vi "УУ.vi"(7 "Func":T1) -> (2 "Read":bool, 3 "Exec":bool, 4 "SelInp":bool, 6 "Wr":bool, 8 "SelOp":bool, 10 "ALU func":T1, 14 "Cread":bool, 15 "ClearAcc":bool)   [LabVIEW 2013]
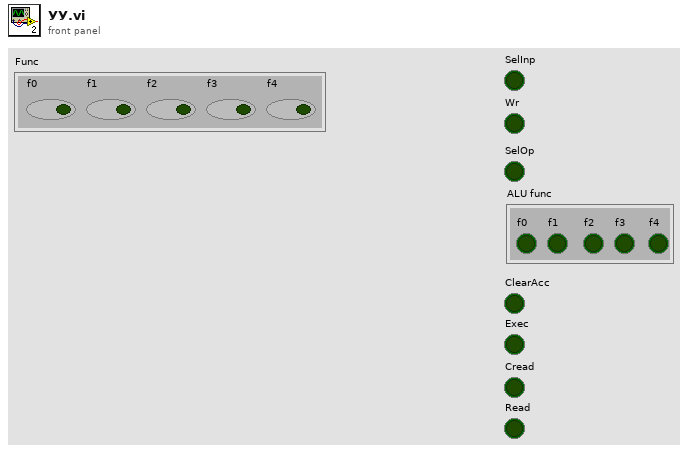
[diagram p1: front panel]
types:
  T1 = cluster{"f0":bool, "f1":bool, "f2":bool, "f3":bool, "f4":bool}
  T2 = cluster{bool, bool, bool, cluster{bool, bool, bool, bool, bool}, bool, bool, bool, bool}
  T3 = cluster{"SelInp":bool, "Wr":bool, "SelOp":bool, "ALU func":cluster{"f0":bool, "f1":bool, "f2":bool, "f3":bool, "f4":bool}, "ClearAcc":bool, "Exec":bool, "Cread":bool, "Read":bool}
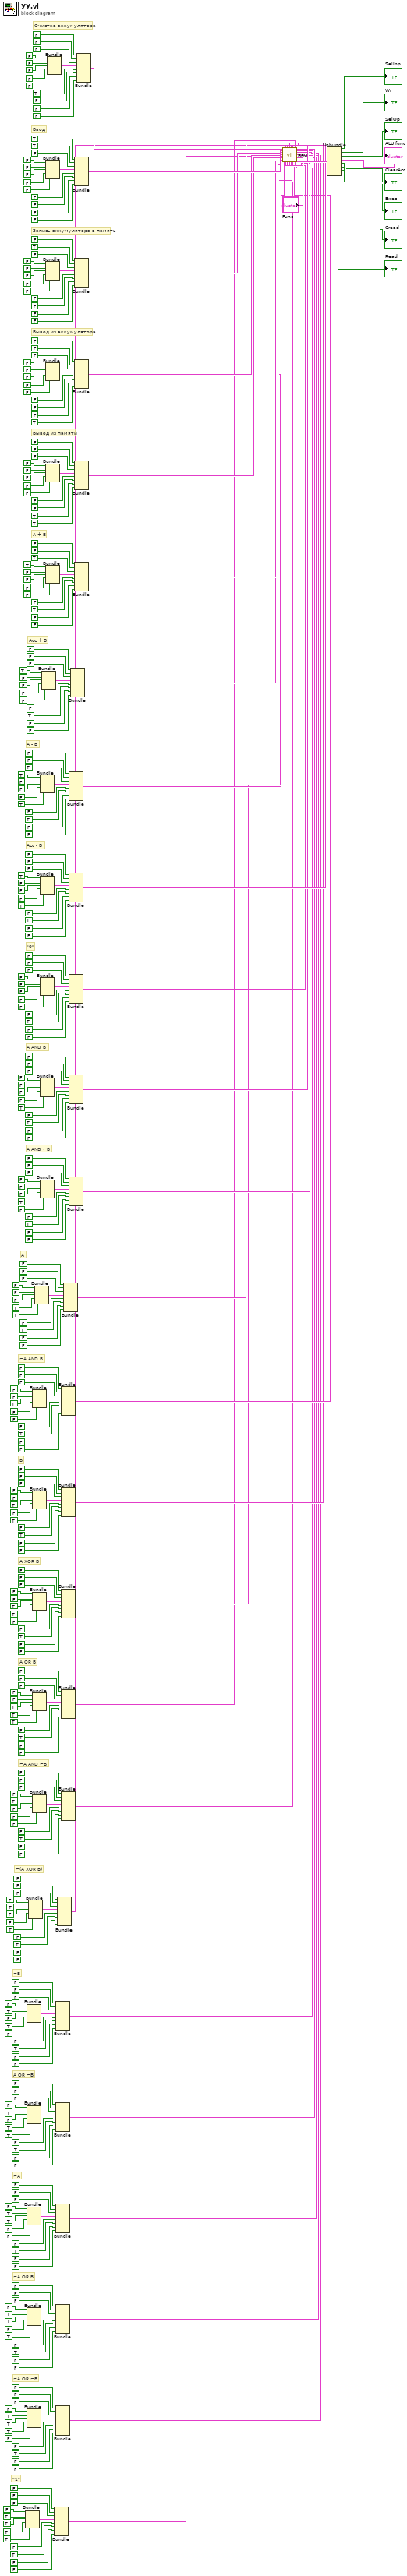
[diagram p0: block diagram]
diagram:
  # "\"1\""
  # "~A OR ~B"
  # "~A OR B"
  # "~A"
  # "A OR ~B"
  # "~B"
  # "~(A XOR B)"
  # "~A AND ~B"
  # "A OR B"
  # "A XOR B"
  # "B"
  # "~A AND B"
  # "A"
  # "A AND ~B"
  # "A AND B"
  # "\"0\""
  # "Acc - B"
  # "A - B"
  # "Acc + B"
  # "A + B"
  # "Вывод из памяти"
  # "Вывод из аккумулятора"
  # "Запись аккумулятора в память"
  # "Ввод"
  # "Очистка аккумулятора"
  n1 = Bundle(FALSE, TRUE, TRUE, TRUE, TRUE) -> (w30:cluster{bool, bool, bool, bool, bool})  [unwired: 1 in]
  n2 = Bundle(FALSE, TRUE, FALSE, TRUE, FALSE) -> (w95:cluster{bool, bool, bool, bool, bool})  [unwired: 1 in]
  n3 = Bundle(FALSE, TRUE, FALSE, TRUE, TRUE) -> (w82:cluster{bool, bool, bool, bool, bool})  [unwired: 1 in]
  n4 = Bundle(FALSE, TRUE, TRUE, FALSE, FALSE) -> (w69:cluster{bool, bool, bool, bool, bool})  [unwired: 1 in]
  n5 = Bundle(FALSE, TRUE, TRUE, FALSE, TRUE) -> (w56:cluster{bool, bool, bool, bool, bool})  [unwired: 1 in]
  n6 = Bundle(FALSE, TRUE, TRUE, TRUE, FALSE) -> (w43:cluster{bool, bool, bool, bool, bool})  [unwired: 1 in]
  n7 = Bundle(FALSE, TRUE, FALSE, FALSE, TRUE) -> (w108:cluster{bool, bool, bool, bool, bool})  [unwired: 1 in]
  n8 = Bundle(FALSE, FALSE, TRUE, FALSE, FALSE) -> (w173:cluster{bool, bool, bool, bool, bool})  [unwired: 1 in]
  n9 = Bundle(FALSE, FALSE, TRUE, FALSE, TRUE) -> (w160:cluster{bool, bool, bool, bool, bool})  [unwired: 1 in]
  n10 = Bundle(FALSE, FALSE, TRUE, TRUE, FALSE) -> (w147:cluster{bool, bool, bool, bool, bool})  [unwired: 1 in]
  n11 = Bundle(FALSE, FALSE, TRUE, TRUE, TRUE) -> (w134:cluster{bool, bool, bool, bool, bool})  [unwired: 1 in]
  n12 = Bundle(FALSE, TRUE, FALSE, FALSE, FALSE) -> (w121:cluster{bool, bool, bool, bool, bool})  [unwired: 1 in]
  n13 = Bundle(FALSE, FALSE, FALSE, TRUE, TRUE) -> (w186:cluster{bool, bool, bool, bool, bool})  [unwired: 1 in]
  n14 = Bundle(TRUE, FALSE, FALSE, FALSE, TRUE) -> (w251:cluster{bool, bool, bool, bool, bool})  [unwired: 1 in]
  n15 = Bundle(TRUE, FALSE, FALSE, FALSE, TRUE) -> (w238:cluster{bool, bool, bool, bool, bool})  [unwired: 1 in]
  n16 = Bundle(FALSE, FALSE, FALSE, FALSE, FALSE) -> (w225:cluster{bool, bool, bool, bool, bool})  [unwired: 1 in]
  n17 = Bundle(FALSE, FALSE, FALSE, FALSE, TRUE) -> (w212:cluster{bool, bool, bool, bool, bool})  [unwired: 1 in]
  n18 = Bundle(FALSE, FALSE, FALSE, TRUE, FALSE) -> (w199:cluster{bool, bool, bool, bool, bool})  [unwired: 1 in]
  n19 = Bundle(TRUE, FALSE, FALSE, FALSE, FALSE) -> (w264:cluster{bool, bool, bool, bool, bool})  [unwired: 1 in]
  n20 = Bundle(FALSE, FALSE, FALSE, FALSE, FALSE) -> (w329:cluster{bool, bool, bool, bool, bool})  [unwired: 1 in]
  n21 = Bundle(FALSE, FALSE, FALSE, FALSE, FALSE) -> (w316:cluster{bool, bool, bool, bool, bool})  [unwired: 1 in]
  n22 = Bundle(FALSE, FALSE, FALSE, FALSE, FALSE) -> (w303:cluster{bool, bool, bool, bool, bool})  [unwired: 1 in]
  n23 = Bundle(FALSE, FALSE, FALSE, FALSE, FALSE) -> (w290:cluster{bool, bool, bool, bool, bool})  [unwired: 1 in]
  n24 = Bundle(TRUE, FALSE, FALSE, FALSE, FALSE) -> (w277:cluster{bool, bool, bool, bool, bool})  [unwired: 1 in]
  n25 = Bundle(FALSE, FALSE, FALSE, FALSE, FALSE) -> (w342:cluster{bool, bool, bool, bool, bool})  [unwired: 1 in]
  n26 = Bundle(FALSE, FALSE, FALSE, w30, FALSE, TRUE, FALSE, FALSE) -> (w1:T2)  [unwired: 1 in]
  n27 = Bundle(FALSE, FALSE, FALSE, w95, FALSE, TRUE, FALSE, FALSE) -> (w6:T2)  [unwired: 1 in]
  n28 = Bundle(FALSE, FALSE, FALSE, w82, FALSE, TRUE, FALSE, FALSE) -> (w5:T2)  [unwired: 1 in]
  n29 = Bundle(FALSE, FALSE, FALSE, w69, FALSE, TRUE, FALSE, FALSE) -> (w4:T2)  [unwired: 1 in]
  n30 = Bundle(FALSE, FALSE, FALSE, w56, FALSE, TRUE, FALSE, FALSE) -> (w3:T2)  [unwired: 1 in]
  n31 = Bundle(FALSE, FALSE, FALSE, w43, FALSE, TRUE, FALSE, FALSE) -> (w2:T2)  [unwired: 1 in]
  n32 = Bundle(FALSE, FALSE, FALSE, w108, FALSE, TRUE, FALSE, FALSE) -> (w7:T2)  [unwired: 1 in]
  n33 = Bundle(FALSE, FALSE, FALSE, w173, FALSE, TRUE, FALSE, FALSE) -> (w12:T2)  [unwired: 1 in]
  n34 = Bundle(FALSE, FALSE, FALSE, w160, FALSE, TRUE, FALSE, FALSE) -> (w11:T2)  [unwired: 1 in]
  n35 = Bundle(FALSE, FALSE, FALSE, w147, FALSE, TRUE, FALSE, FALSE) -> (w10:T2)  [unwired: 1 in]
  n36 = Bundle(FALSE, FALSE, FALSE, w134, FALSE, TRUE, FALSE, FALSE) -> (w9:T2)  [unwired: 1 in]
  n37 = Bundle(FALSE, FALSE, FALSE, w121, FALSE, TRUE, FALSE, FALSE) -> (w8:T2)  [unwired: 1 in]
  n38 = Bundle(FALSE, FALSE, FALSE, w186, FALSE, TRUE, FALSE, FALSE) -> (w13:T2)  [unwired: 1 in]
  n39 = Bundle(FALSE, FALSE, TRUE, w251, FALSE, TRUE, FALSE, FALSE) -> (w18:T2)  [unwired: 1 in]
  n40 = Bundle(FALSE, FALSE, FALSE, w238, FALSE, TRUE, FALSE, FALSE) -> (w17:T2)  [unwired: 1 in]
  n41 = Bundle(FALSE, FALSE, FALSE, w225, FALSE, TRUE, FALSE, FALSE) -> (w16:T2)  [unwired: 1 in]
  n42 = Bundle(FALSE, FALSE, FALSE, w212, FALSE, TRUE, FALSE, FALSE) -> (w15:T2)  [unwired: 1 in]
  n43 = Bundle(FALSE, FALSE, FALSE, w199, FALSE, TRUE, FALSE, FALSE) -> (w14:T2)  [unwired: 1 in]
  n44 = Bundle(FALSE, FALSE, FALSE, w264, FALSE, TRUE, FALSE, FALSE) -> (w19:T2)  [unwired: 1 in]
  n45 = Bundle(TRUE, TRUE, FALSE, w329, FALSE, FALSE, FALSE, FALSE) -> (w24:T2)  [unwired: 1 in]
  n46 = Bundle(FALSE, TRUE, FALSE, w316, FALSE, FALSE, FALSE, FALSE) -> (w23:T2)  [unwired: 1 in]
  n47 = Bundle(FALSE, FALSE, FALSE, w303, FALSE, FALSE, FALSE, TRUE) -> (w22:T2)  [unwired: 1 in]
  n48 = Bundle(FALSE, FALSE, FALSE, w290, FALSE, FALSE, TRUE, TRUE) -> (w21:T2)  [unwired: 1 in]
  n49 = Bundle(FALSE, FALSE, TRUE, w277, FALSE, TRUE, FALSE, FALSE) -> (w20:T2)  [unwired: 1 in]
  n50 = Bundle(FALSE, FALSE, FALSE, w342, TRUE, FALSE, FALSE, FALSE) -> (w25:T2)  [unwired: 1 in]
  n51 = call "BFM.vi"("in 0"=w25, "in 1"=w24, "in 2"=w23, "in 3"=w22, "in 4"=w21, "in 5"=w20, "in 6"=w19, "in 7"=w18, "in 8"=w17, "in 9"=w16, "in 10"=w15, "in 11"=w14, "in 12"=w13, "in 13"=w12, "in 14"=w11, "in 15"=w10, "in 16"=w9, "in 17"=w8, "in 18"=w7, "in 19"=w6, "in 20"=w5, "in 21"=w4, "in 22"=w3, "in 23"=w2, "in 24"=w1, "Func"="Func") -> ("out"=w360:T3)  [unwired: 1 in]
  n52 = Unbundle(w360) -> ("SelInp"=→"SelInp":bool, "Wr"=→"Wr":bool, "SelOp"=→"SelOp":bool, "ALU func"=→"ALU func":T1, "ClearAcc"=→"ClearAcc":bool, "Exec"=→"Exec":bool, "Cread"=→"Cread":bool, "Read"=→"Read":bool)
